vi "Read WriteTimeout.vi"(8 "error in (no error)":errorcluster, 11 "TcpSocket in":refnum<class "TcpSocket.lvclass">) -> (0 "error out":errorcluster, 2 "WriteTimeout":i32=5000, 3 "TcpSocket out":refnum<class "TcpSocket.lvclass">)   [LabVIEW 2021, in "TcpSocket.lvlib" / "TcpSocket.lvclass"]
uses:
  TcpSocket.lvclass
  TcpSocket.lvclass/TcpSocket.ctl
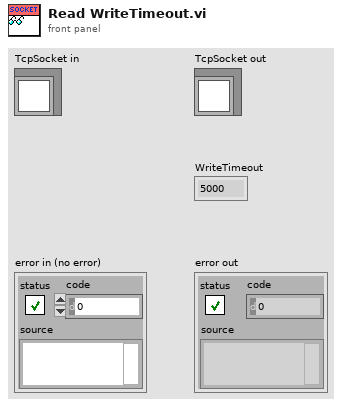
[diagram p1: front panel]
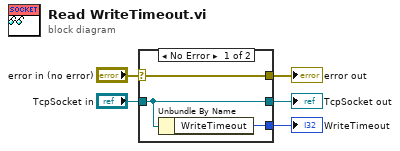
[diagram p0: block diagram]
diagram:
  n1 = case shown="No Error" "error in (no error)" {
    selector: "error in (no error)" -> [w8 w9]
    tunnel: [w8 w9] -> w4
    tunnel: [w7 w10] -> w2
    tunnel: "TcpSocket in" -> [w7 w10]
    tunnel: [w6 _] -> w1
    frame No Error {
      n2 = Unbundle By Name(w7) -> ("WriteTimeout"=w6:i32)
    }
    frame Error {
    }
  }
  "error out" <- w4
  "TcpSocket out" <- w2
  "WriteTimeout" <- w1
